vi "主界面.vi"() -> ()   [LabVIEW 2014]
panel:
  out "字符串":string
  out "选项卡控件":T1
  out "修读学院：":string caption="学号："
  out "修读专业：":string caption="学号："
  out "入学年份：":string caption="学号："
  out "学习信息":string caption="学生姓名："
  out "基本信息":string caption="学生姓名："
  out "学号： 2":string caption="学号："
  out "学生姓名： 2":string caption="学生姓名："
  out "性别：":string caption="学号："
  out "民族：":string caption="学号："
  out "生日：":string caption="学号："
  in  "实验讲义查看":refnum<k7>(container) caption="网页浏览器"
  in  "使用帮助查看":refnum<k7>(container) caption="网页浏览器"
  in  "实验内容":bool
  in  "退出平台":bool
  in  "使用帮助":bool
  in  "查看讲义":bool
  in  "用户信息":bool
  in  "仪器面板":bool
  in  "连接仪器":bool
  out "仪器状态：":string
  out "学号：":string
  out "学生姓名：":string
  out "学习时间：":string
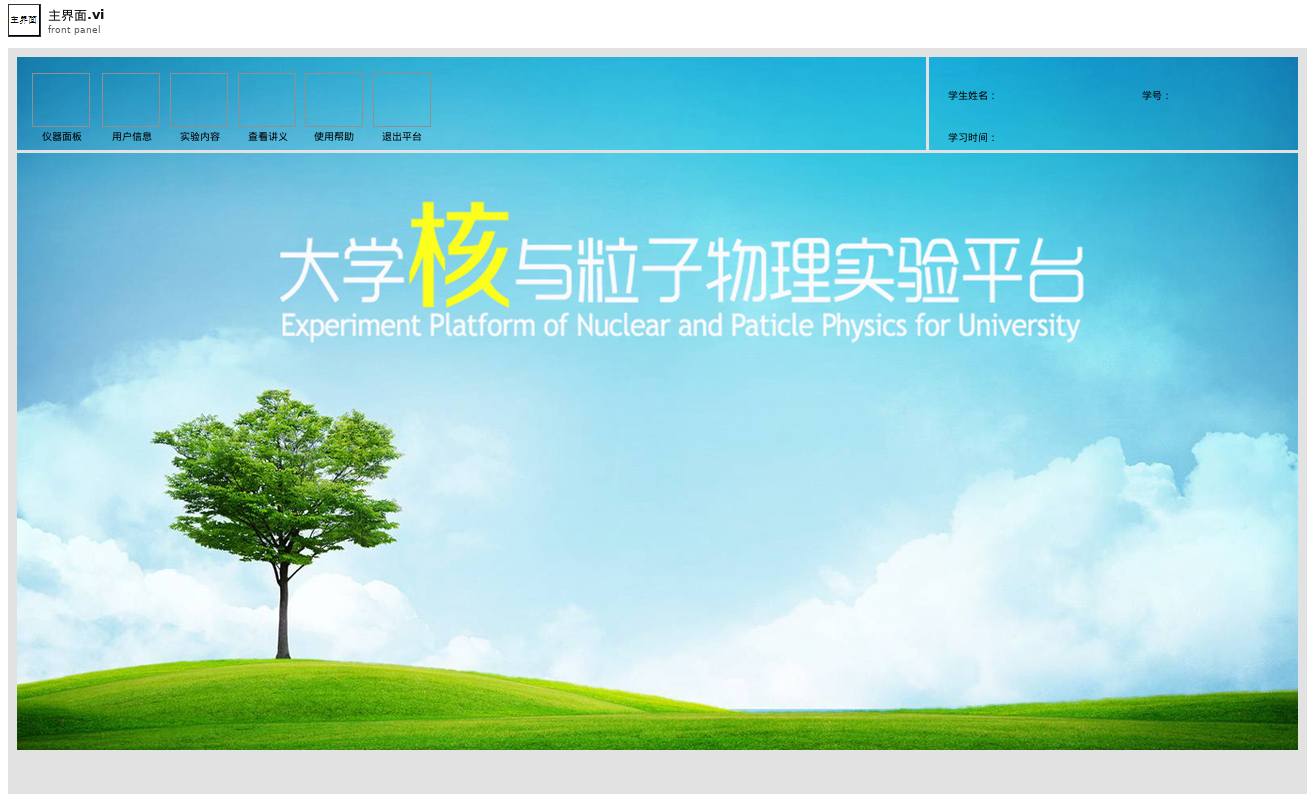
[diagram p1: front panel]
types:
  T1 = typedef "主界面_透明选项卡.ctl" = enum32{"欢迎界面", "连接仪器 ", "仪器面板  ", "用户信息", "实验内容", "查看讲义", "使用帮助", "退出平台"}
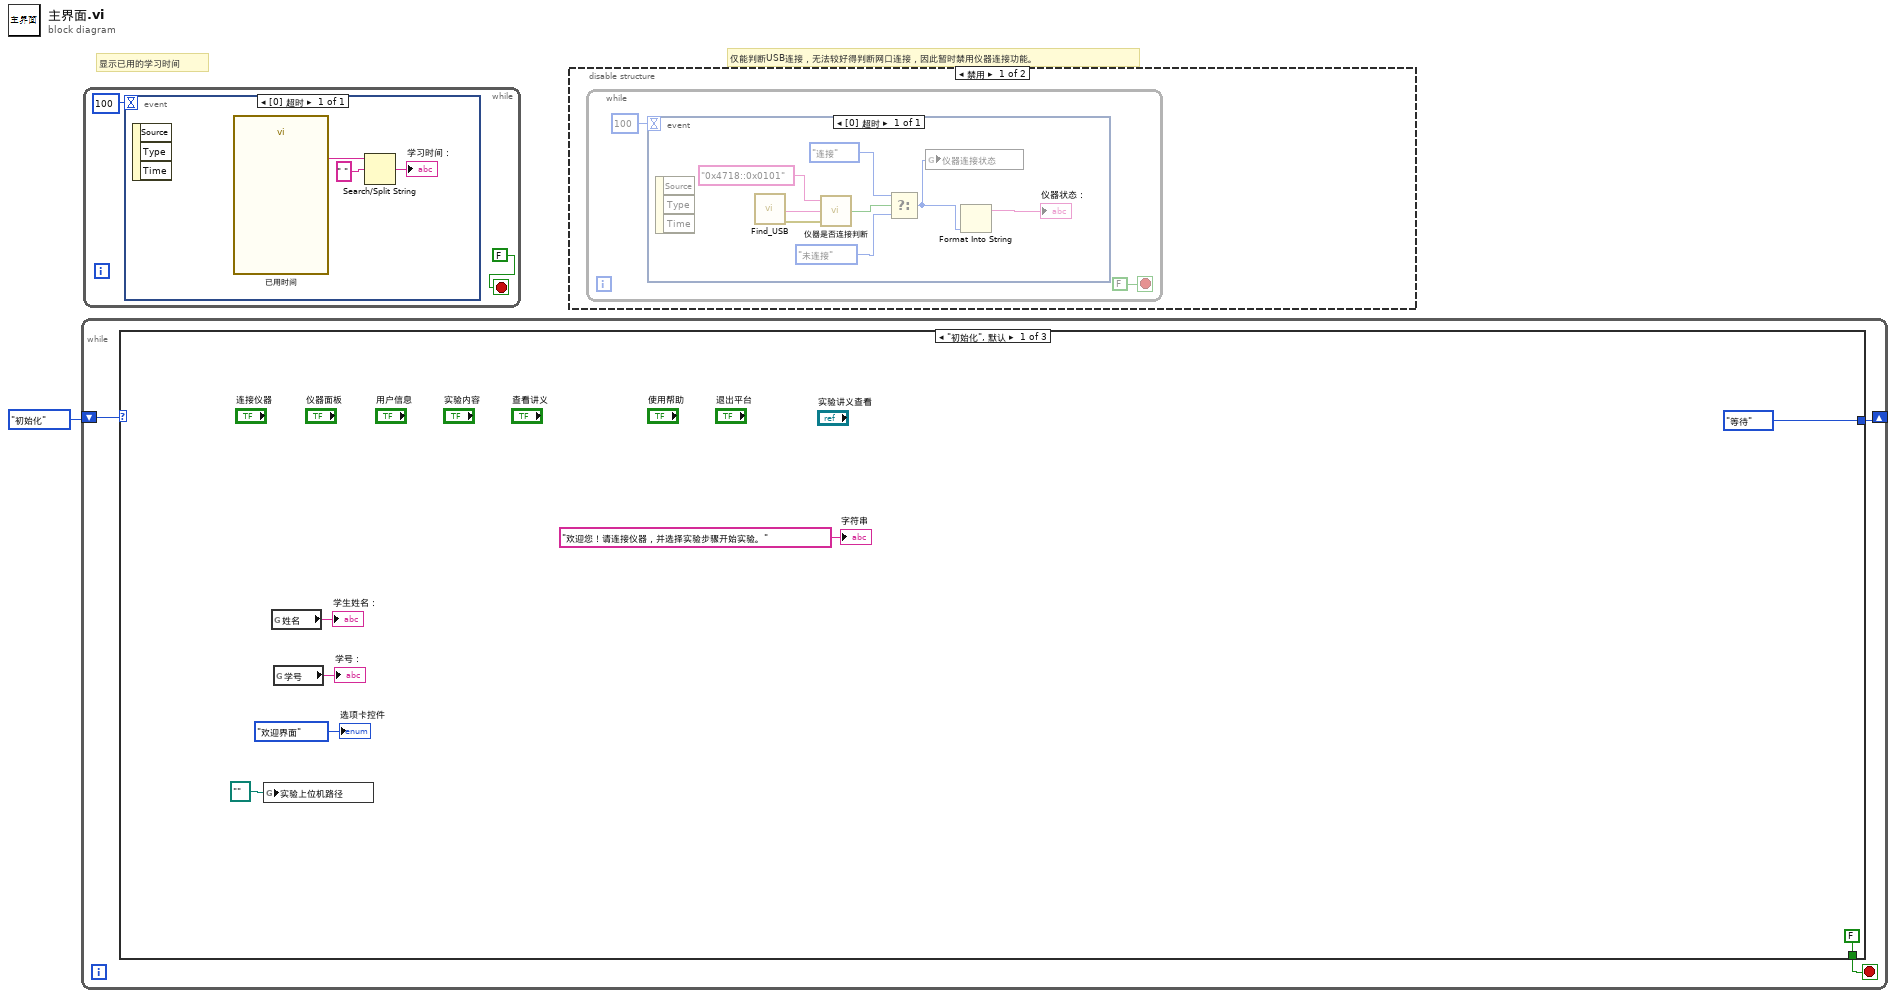
[diagram p0: block diagram]
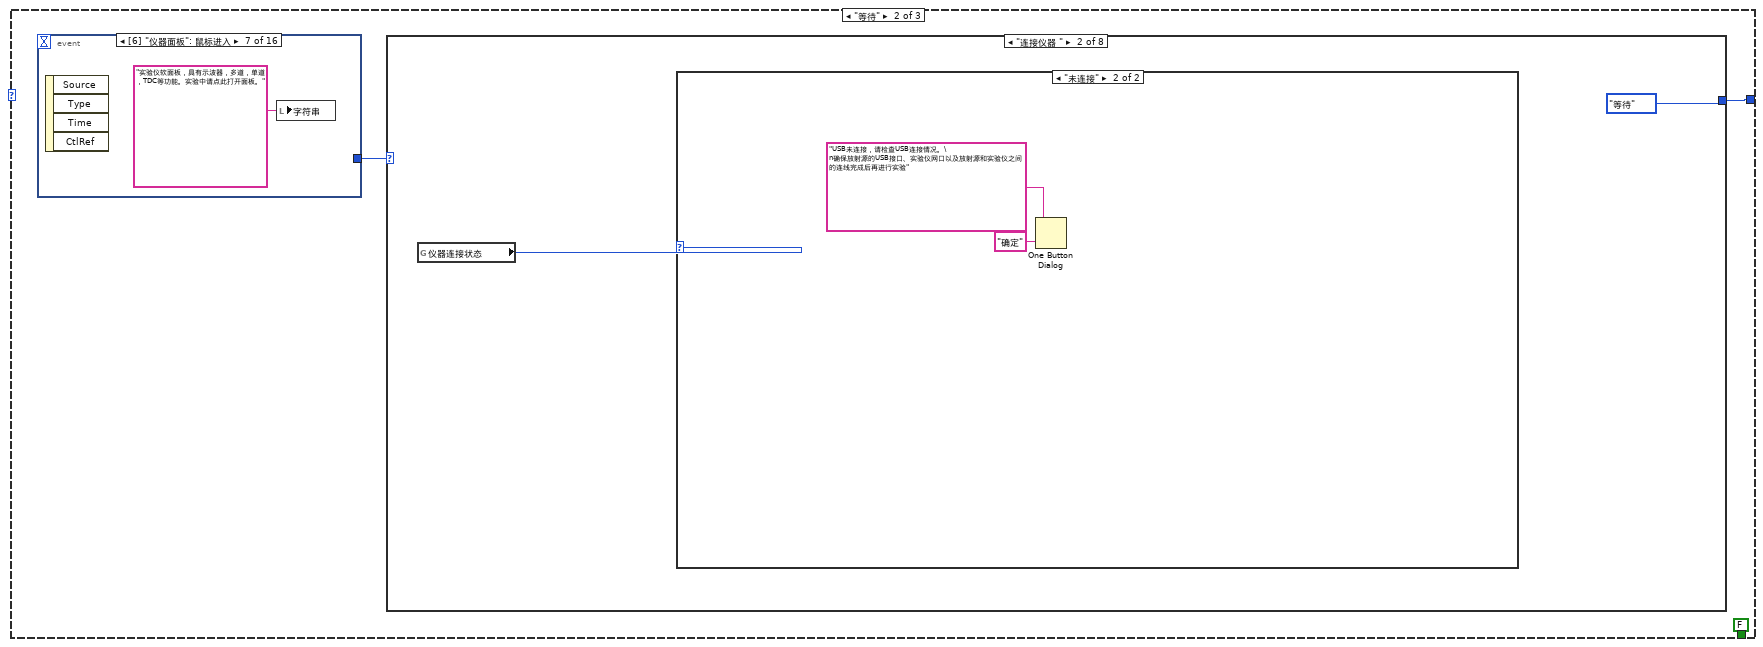
[diagram p3: hidden frame]
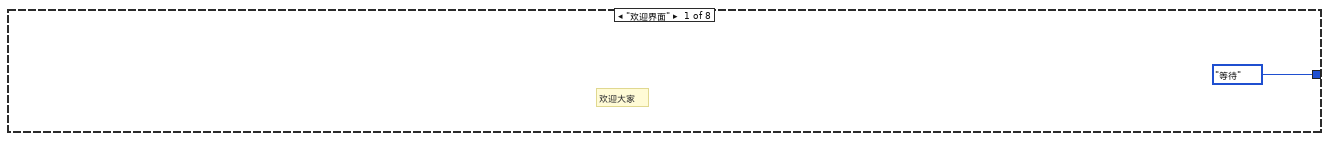
[diagram p4: hidden frame]
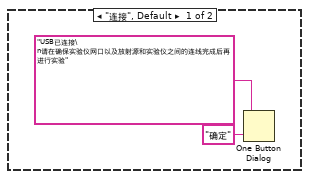
[diagram p5: hidden frame]
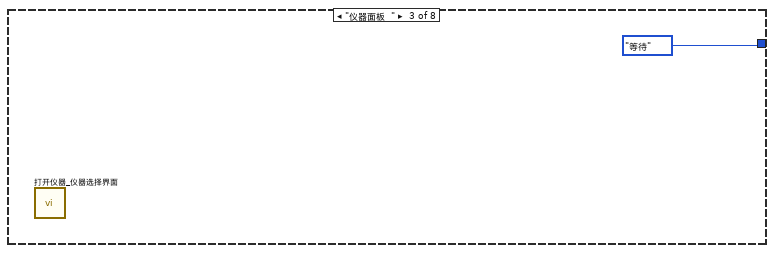
[diagram p6: hidden frame]
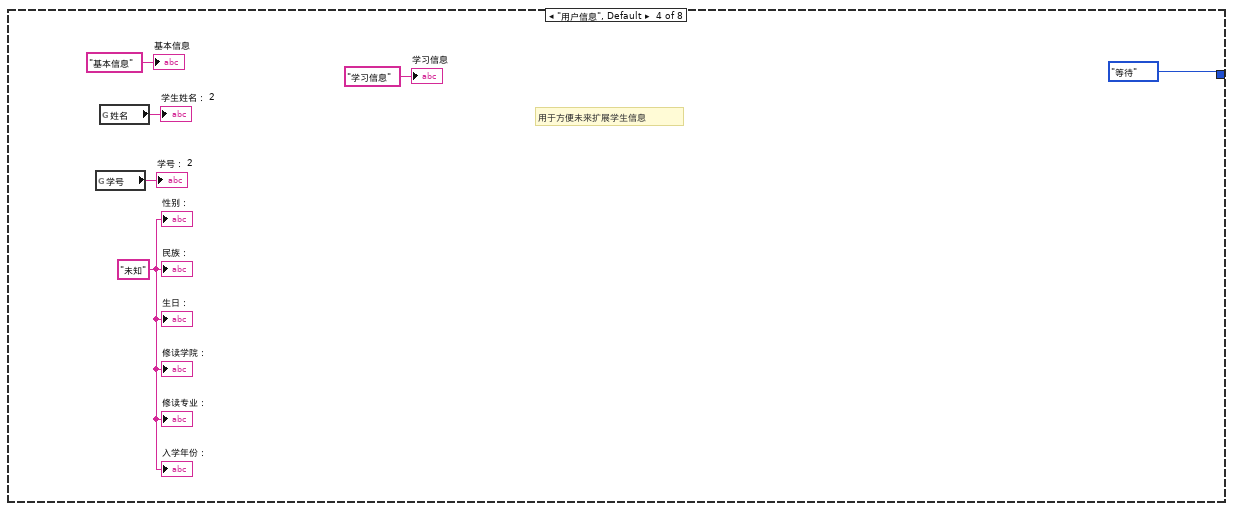
[diagram p7: hidden frame]
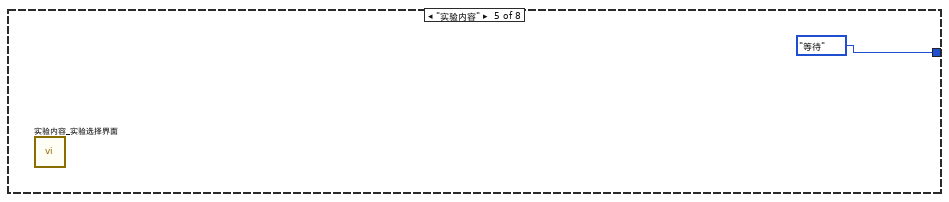
[diagram p8: hidden frame]
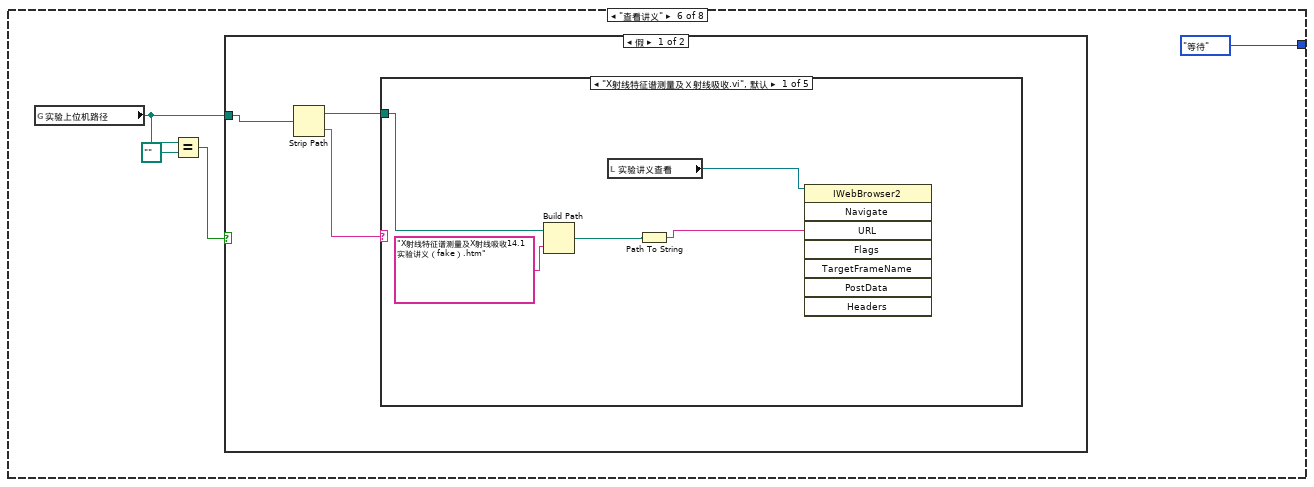
[diagram p9: hidden frame]
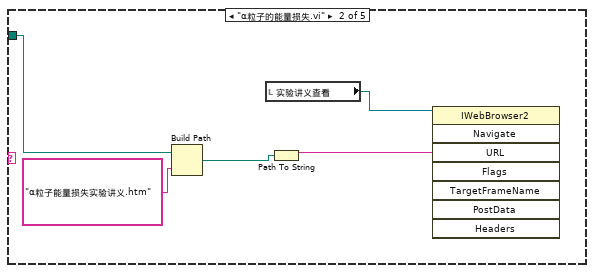
[diagram p10: hidden frame]
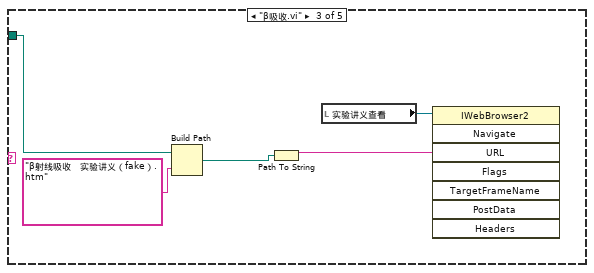
[diagram p11: hidden frame]
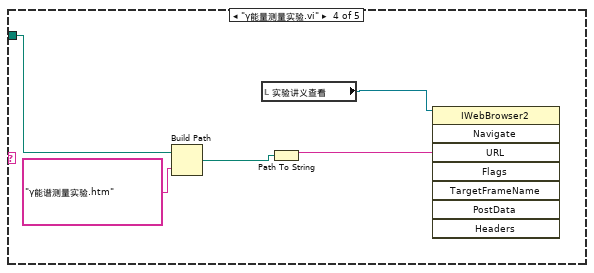
[diagram p12: hidden frame]
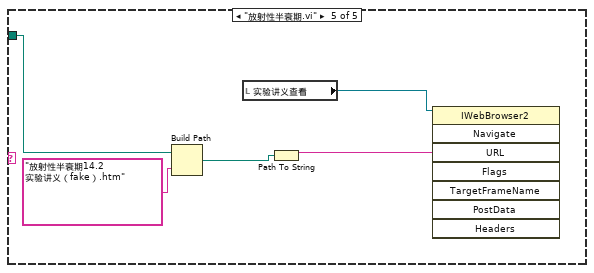
[diagram p13: hidden frame]
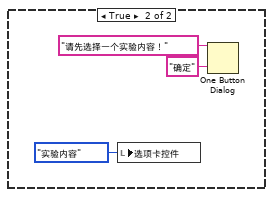
[diagram p14: hidden frame]
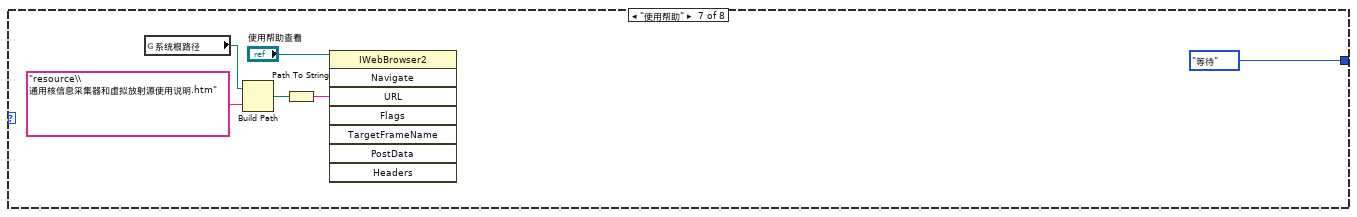
[diagram p15: hidden frame]
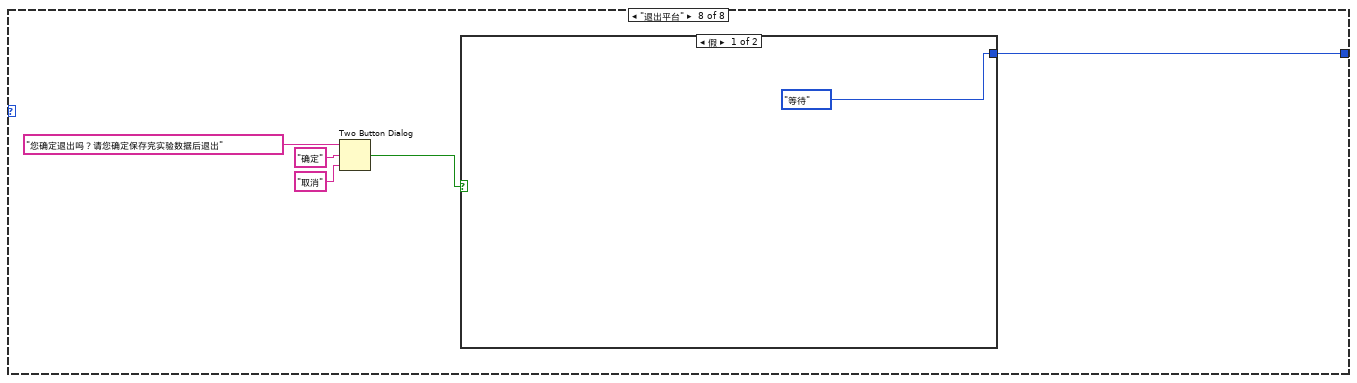
[diagram p16: hidden frame]
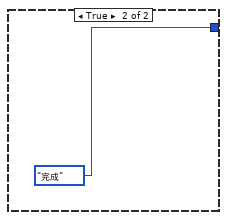
[diagram p17: hidden frame]
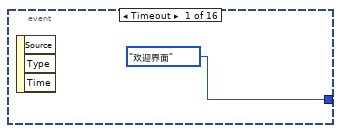
[diagram p18: hidden frame]
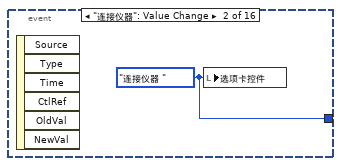
[diagram p19: hidden frame]
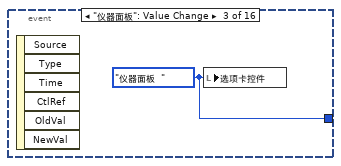
[diagram p20: hidden frame]
diagram:
  # "仅能判断USB连接，无法较好得判断网口连接，因此暂时禁用仪器连接功能。"
  # "显示已用的学习时间"
  n1 = while {
    shift-right: [w3] -> _
    shift-left: enum16{"初始化", "等待", "完成"}."初始化" -> [w4]
    stop <- w2 stop-if-true
    n2 = case shown="\"初始化\", 默认" w4 {
      tunnel: [enum16{"初始化", "等待", "完成"}."等待" w13 enum16{"初始化", "等待", "完成"}."完成"] -> w3
      tunnel: [FALSE FALSE w94] -> w2
      frame "初始化", Default {
        n3 = global write "系统全局变量.vi" "实验上位机路径"(path "" ("实验上位机路径")) -> ()
        n4 = global read "系统全局变量.vi" "姓名"() -> (→"学生姓名：":string)
        n5 = global read "系统全局变量.vi" "学号"() -> (→"学号：":string)
        "选项卡控件" <- 主界面_透明选项卡."欢迎界面" ("选项卡控件")
        "字符串" <- "欢迎您！请连接仪器，并选择实验步骤开始实验。" ("字符串")
      }
      frame "等待" {
        n6 = event shown="[6] \"仪器面板\": 鼠标进入" {
          selector: _ -> [_ _ _ _ _ _ _ _ _ _ _ _ _ _ _ _]
          dyn-events: _ -> [_ _ _ _ _ _ _ _ _ _ _ _ _ _ _ _]
          timeout: _ -> [_ _ _ _ _ _ _ _ _ _ _ _ _ _ _ _]
          tunnel: [主界面_透明选项卡."欢迎界面" ("选项卡控件") w79 w80 w81 w82 _ _ _ _ _ _ _ _ w91 w92 w93] -> w12
          event Timeout {
            n7 = event-data() -> ()  [unwired: 1 in, 3 out]
          }
          event "连接仪器": Value Change {
            w79 = 主界面_透明选项卡."连接仪器 " ("选项卡控件")
            n8 = event-data() -> ()  [unwired: 1 in, 6 out]
            n9 = local write "选项卡控件"(w79) -> ()
          }
          event "仪器面板": Value Change {
            w80 = 主界面_透明选项卡."仪器面板  " ("选项卡控件")
            n10 = event-data() -> ()  [unwired: 1 in, 6 out]
            n11 = local write "选项卡控件"(w80) -> ()
          }
          event "用户信息": Value Change {
            w81 = 主界面_透明选项卡."用户信息" ("选项卡控件")
            n12 = event-data() -> ()  [unwired: 1 in, 6 out]
            n13 = local write "选项卡控件"(w81) -> ()
          }
          event "实验内容": Value Change {
            w82 = 主界面_透明选项卡."实验内容" ("选项卡控件")
            n14 = event-data() -> ()  [unwired: 1 in, 6 out]
            n15 = local write "选项卡控件"(w82) -> ()
          }
          event "连接仪器": Mouse Enter {
            n16 = event-data() -> ()  [unwired: 1 in, 4 out]
            n17 = local write "字符串"("通过USB连接核与粒子物理实验仪。请在实验开始前完成此步骤。" ("字符串")) -> ()
          }
          event "仪器面板": Mouse Enter {
            n18 = event-data() -> ()  [unwired: 1 in, 4 out]
            n19 = local write "字符串"("实验仪软面板，具有示波器，多道，单道，TDC等功能。实验中请点此打开面板。" ("字符串")) -> ()
          }
          event "用户信息": Mouse Enter {
            n20 = event-data() -> ()  [unwired: 1 in, 4 out]
            n21 = local write "字符串"("显示当前用户的基本资料。" ("字符串")) -> ()
          }
          event "查看讲义": Mouse Enter {
            n22 = event-data() -> ()  [unwired: 1 in, 4 out]
            n23 = local write "字符串"("查看当前实验的实验讲义，请先选择实验内容后再查看。" ("字符串")) -> ()
          }
          event "使用帮助": Mouse Enter {
            n24 = event-data() -> ()  [unwired: 1 in, 4 out]
            n25 = local write "字符串"("查看本实验平台的帮助文档。对平台的使用存在任何疑惑请立即使用此功能。" ("字符串")) -> ()
          }
          event "退出平台": Mouse Enter {
            n26 = event-data() -> ()  [unwired: 1 in, 4 out]
            n27 = local write "字符串"("退出平台，结束本次实验。请在退出时注意保存实验数据，以免丢失。" ("字符串")) -> ()
          }
          event "连接仪器", "仪器面板", "用户信息", "查看讲义", "使用帮助", "退出平台", "实验内容": Mouse Leave {
            n28 = event-data() -> ()  [unwired: 1 in, 4 out]
            n29 = local write "字符串"("欢迎您！请连接仪器，并选择实验步骤开始实验。" ("字符串")) -> ()
          }
          event "实验内容": Mouse Enter {
            n30 = event-data() -> ()  [unwired: 1 in, 4 out]
            n31 = local write "字符串"("选择要进行的实验，完成此步骤后可查看相应的实验讲义" ("字符串")) -> ()
          }
          event "查看讲义": Value Change {
            w91 = 主界面_透明选项卡."查看讲义" ("选项卡控件")
            n32 = event-data() -> ()  [unwired: 1 in, 6 out]
            n33 = local write "选项卡控件"(w91) -> ()
          }
          event "使用帮助": Value Change {
            w92 = 主界面_透明选项卡."使用帮助" ("选项卡控件")
            n34 = event-data() -> ()  [unwired: 1 in, 6 out]
            n35 = local write "选项卡控件"(w92) -> ()
          }
          event "退出平台": Value Change {
            w93 = 主界面_透明选项卡."退出平台" ("选项卡控件")
            n36 = event-data() -> ()  [unwired: 1 in, 6 out]
            n37 = local write "选项卡控件"(w93) -> ()
          }
        }
        n38 = case shown="\"连接仪器 \"" w12 {
          tunnel: [enum16{"初始化", "等待", "完成"}."等待" enum16{"初始化", "等待", "完成"}."等待" enum16{"初始化", "等待", "完成"}."等待" enum16{"初始化", "等待", "完成"}."等待" enum16{"初始化", "等待", "完成"}."等待" enum16{"初始化", "等待", "完成"}."等待" enum16{"初始化", "等待", "完成"}."等待" w75] -> w13
          frame "欢迎界面" {
            # "欢迎大家"
          }
          frame "连接仪器 " {
            n39 = global read "系统全局变量.vi" "仪器连接状态"() -> (w16:enum16{"连接", "未连接"})
            n40 = case shown="\"未连接\"" w16 {
              frame "连接", Default {
                n41 = One Button Dialog(message="USB已连接\n请在确保实验仪网口以及放射源和实验仪之间的连线完成后再进行实验" ("消息"), button name ("OK")="确定" ("按钮名称（“确定”）")) -> ()  [unwired: 1 out]
              }
              frame "未连接" {
                n42 = One Button Dialog(message="USB未连接，请检查USB连接情况。\n确保放射源的USB接口、实验仪网口以及放射源和实验仪之间的连线完成后再进行实验" ("消息"), button name ("OK")="确定" ("按钮名称（“确定”）")) -> ()  [unwired: 1 out]
              }
            }
          }
          frame "仪器面板  " {
            n43 = call "打开仪器_仪器选择界面.vi"() -> ()  [unwired: 12 in]
          }
          frame "用户信息", Default {
            w23 = "未知" ("基本信息")
            # "用于方便未来扩展学生信息"
            n44 = global read "系统全局变量.vi" "学号"() -> (→"学号： 2":string)
            n45 = global read "系统全局变量.vi" "姓名"() -> (→"学生姓名： 2":string)
            "性别：" <- w23
            "民族：" <- w23
            "生日：" <- w23
            "基本信息" <- "基本信息" ("基本信息")
            "学习信息" <- "学习信息" ("学习信息")
            "入学年份：" <- w23
            "修读专业：" <- w23
            "修读学院：" <- w23
          }
          frame "实验内容" {
            n46 = call "实验内容_实验选择界面.vi"() -> ()  [unwired: 2 in]
          }
          frame "查看讲义" {
            n47 = global read "系统全局变量.vi" "实验上位机路径"() -> (w30:path)
            n48 = Equal?(x=w30, y=path "") -> (x = y?=w31:bool)
            n49 = case shown="假" w31 {
              tunnel: w30 -> [w36 _]
              frame False {
                n50 = Strip Path(path=w36) -> (stripped path=w34:path, name=w35:string)
                n51 = case shown="\"X射线特征谱测量及Ｘ射线吸收.vi\", 默认" w35 {
                  tunnel: w34 -> [w41 w46 w51 w56 w61]
                  frame "X射线特征谱测量及Ｘ射线吸收.vi", Default {
                    n52 = Build Path(base path=w41, name or relative path="X射线特征谱测量及X射线吸收14.1   实验讲义（fake）.htm" ("名称或相对路径")) -> (appended path=w37:path)
                    n53 = local read "实验讲义查看"() -> (w39:refnum<k7>)
                    n54 = Path To String(path=w37) -> (string=w38:string)
                    n55 = invoke class="IWebBrowser2" method="Navigate"(reference=w39, "URL"=w38) -> ()  [unwired: 6 in, 8 out]
                  }
                  frame "α粒子的能量损失.vi" {
                    n56 = Build Path(base path=w46, name or relative path="α粒子能量损失实验讲义.htm" ("名称或相对路径")) -> (appended path=w43:path)
                    n57 = local read "实验讲义查看"() -> (w42:refnum<k7>)
                    n58 = Path To String(path=w43) -> (string=w44:string)
                    n59 = invoke class="IWebBrowser2" method="Navigate"(reference=w42, "URL"=w44) -> ()  [unwired: 6 in, 8 out]
                  }
                  frame "β吸收.vi" {
                    n60 = Build Path(base path=w51, name or relative path="β射线吸收   实验讲义（fake）.htm" ("名称或相对路径")) -> (appended path=w48:path)
                    n61 = Path To String(path=w48) -> (string=w49:string)
                    n62 = local read "实验讲义查看"() -> (w47:refnum<k7>)
                    n63 = invoke class="IWebBrowser2" method="Navigate"(reference=w47, "URL"=w49) -> ()  [unwired: 6 in, 8 out]
                  }
                  frame "γ能量测量实验.vi" {
                    n64 = Build Path(base path=w56, name or relative path="γ能谱测量实验.htm" ("名称或相对路径")) -> (appended path=w53:path)
                    n65 = local read "实验讲义查看"() -> (w52:refnum<k7>)
                    n66 = Path To String(path=w53) -> (string=w54:string)
                    n67 = invoke class="IWebBrowser2" method="Navigate"(reference=w52, "URL"=w54) -> ()  [unwired: 6 in, 8 out]
                  }
                  frame "放射性半衰期.vi" {
                    n68 = Build Path(base path=w61, name or relative path="放射性半衰期14.2   实验讲义（fake）.htm" ("名称或相对路径")) -> (appended path=w58:path)
                    n69 = local read "实验讲义查看"() -> (w57:refnum<k7>)
                    n70 = Path To String(path=w58) -> (string=w59:string)
                    n71 = invoke class="IWebBrowser2" method="Navigate"(reference=w57, "URL"=w59) -> ()  [unwired: 6 in, 8 out]
                  }
                }
              }
              frame True {
                n72 = local write "选项卡控件"(主界面_透明选项卡."实验内容" ("选项卡控件")) -> ()
                n73 = One Button Dialog(message="请先选择一个实验内容！" ("消息"), button name ("OK")="确定" ("按钮名称（“确定”）")) -> ()  [unwired: 1 out]
              }
            }
          }
          frame "使用帮助" {
            n74 = global read "系统全局变量.vi" "系统根路径"() -> (w69:path)
            n75 = Build Path(base path=w69, name or relative path="resource\\通用核信息采集器和虚拟放射源使用说明.htm" ("名称或相对路径")) -> (appended path=w67:path)
            n76 = Path To String(path=w67) -> (string=w66:string)
            n77 = invoke class="IWebBrowser2" method="Navigate"(reference="使用帮助查看", "URL"=w66) -> ()  [unwired: 6 in, 8 out]
          }
          frame "退出平台" {
            n78 = Two Button Dialog(message="您确定退出吗？请您确定保存完实验数据后退出" ("消息"), 1:"取消" ("F按钮名称（“取消”）"), 2:"确定" ("T按钮名称（“确定”）")) -> (T button?=w71:bool)
            n79 = case shown="假" w71 {
              tunnel: [enum16{"初始化", "等待", "完成"}."等待" enum16{"初始化", "等待", "完成"}."完成"] -> w75
              frame False {
              }
              frame True {
              }
            }
          }
        }
      }
      frame "完成" {
        w94 = TRUE
        n80 = Quit LabVIEW(quit? (T)=w94) -> ()
      }
    }
  }
  n81 = while {
    stop <- FALSE stop-if-true
    n82 = event shown="[0] 超时" {
      selector: _ -> [_]
      dyn-events: _ -> [_]
      timeout: 100 -> [_]
      event Timeout {
        n83 = event-data() -> ()  [unwired: 1 in, 3 out]
        n84 = call "已用时间"() -> ("Elapsed Time Text"=w100:string)  [unwired: 12 in, 7 out]
        n85 = Search/Split String(string=w100, search string/char (-)=" " ("搜索字符串/字符(-)")) -> (match + rest of string=→"学习时间：":string)  [unwired: 1 in, 2 out]
      }
    }
  }
  n86 = disable-structure shown="禁用" {
    frame Disabled {
      n87 = while {
        stop <- FALSE stop-if-true
        n88 = event shown="[0] 超时" {
          selector: _ -> [_]
          dyn-events: _ -> [_]
          timeout: 100 -> [_]
          event Timeout {
            n89 = event-data() -> ()  [unwired: 1 in, 3 out]
            n90 = call "Find_USB.vi"() -> ("错误输出"=w109:errorcluster, "元素"=w108:string)  [unwired: 10 in]
            n91 = call "仪器是否连接判断.vi"("错误输入（无错误）"=w109, "元素"=w108, "VIDPID"="0x4718::0x0101" ("y")) -> ("仪器是否连接"=w110:bool)
            n92 = Select(t=enum16{"连接", "未连接"}."连接" ("仪器连接状态"), s=w110, f=enum16{"连接", "未连接"}."未连接" ("仪器连接状态")) -> (s? t:f=w105:enum16{"连接", "未连接"})
            n93 = global write "系统全局变量.vi" "仪器连接状态"(w105) -> ()
            n94 = Format Into String(w105) -> (resulting string=→"仪器状态：":string)  [unwired: 3 in, 1 out]
          }
        }
      }
    }
    frame Enabled {
    }
  }
